vi "Main Page.vi"(8 "error in (no error)":errorcluster, 11 "Node Ptr":T3 format="%.0x") -> (0 "error out":errorcluster)   [LabVIEW 2020, in "Instrument Addon System Explorer.lvlib"]
uses:
  Instrument Addon System Explorer.lvlib
  <vilib>/NI VeriStand/Custom Device API/Custom Device Item Ref.ctl
  Addon Shared/Types/FG Control.ctl
  <vilib>/NI/NI VeriStand Hardware Resource Discovery/_Types/Filter Type.ctl
  <vilib>/NI/NI VeriStand Advanced SysDef API/SysDef API/SysDef.Property.Get.vi
  <vilib>/NI/NI VeriStand Advanced SysDef API/_SubVIs/SysDef.Property.Get.String.vi
  <vilib>/NI/NI VeriStand Advanced SysDef API/SysDef API/SysDef.Property.Set.vi
  <vilib>/NI/NI VeriStand Advanced SysDef API/_SubVIs/SysDef.Property.Set.String.vi
  <vilib>/NI VeriStand/Custom Device API/NI VeriStand - Get Item Property.vi
  <vilib>/NI VeriStand/Custom Device API/Get Item Property (Boolean).vi
  <vilib>/NI VeriStand/Custom Device API/Get Item Property (U32).vi
  <vilib>/NI VeriStand/Custom Device API/Get Item Property (String).vi
  <vilib>/NI VeriStand/Custom Device API/NI VeriStand - Set Item Property.vi
  <vilib>/NI VeriStand/Custom Device API/Set Item Property (Boolean).vi
  <vilib>/NI VeriStand/Custom Device API/Set Item Property (U32).vi
  <vilib>/NI VeriStand/Custom Device API/Set Item Property (String).vi
  <vilib>/Utility/LVClass/Get LV Class Default Value.vi
  Includes/Protocols.lvlibp/Protocol Parent/Protocol Parent.lvclass
  <vilib>/NI VeriStand/Custom Device API/Custom Device API.lvlib
  Addon Shared/Instrument Addon Shared.lvlib
  <vilib>/NI/NI VeriStand Hardware Resource Discovery/NIVS Hardware Discovery.lvlib
  APIs/Scripting API/Instrument Addon Scripting API.lvlib
panel:
  out "Version":string
  in  "PCL Decimation":u32=1 min=1 max=10000 step=1
  in  "Protocol Settings":T1(tab)=enum."TCP/IP"
  in  "COM Browse":bool
  in  "Termination Character":u8=10 format="%.0x"
  in  "End Write":bool=TRUE caption="End Write on Termination Character?"
  in  "End Read":bool=TRUE caption="End Read on Termination Character?"
  in  "XOFF":T2(ring)=enum."DC3"
  in  "XON":T2(ring)=enum."DC1"
  in  "Flow Control":u16(ring) items=["None"=0, "XON/XOFF"=1, "RTS/CTS"=2, "DTR/DSR"=4]
  in  "Stop Bits":u16(ring)=10 items=["1.0"=10, "1.5"=15, "2.0"=20]
  in  "Parity":enum16{"None", "Odd", "Even", "Mark", "Space"}(ring)
  in  "Data Bits":u16=8 min=5 max=8 step=1
  in  "Baud Rate":u32(ring)=9600 items=["75"=75, "110"=110, "134"=134, "150"=150, "300"=300, "600"=600, "1200"=1200, "1800"=1800, "2400"=2400, "4800"=4800, "7200"=7200, "9600"=9600, "14400"=14400, "19200"=19200, "28800"=28800, "38400"=38400, "56000"=56000, "57600"=57600, "115200"=115200, "128000"=128000, "230400"=230400, "460800"=460800, "921600"=921600, "1843200"=1843200, "3000000"=3000000]
  in  "Port":string="COM1"
  in  "VISA Browse":bool
  in  "Append Write Termination Character":bool caption="Append Write Termination Character?"
  in  "Timeout":u32=2000 caption="Timeout (ms)"
  in  "Termination Character":u8=10 format="%.0x"
  in  "Enable Termination Character":bool=TRUE caption="Enable Termination Character?"
  in  "VISA Resource":string="GPIB0::2::INSTR"
  in  "Port":u16
  in  "IP Address":string="localhost"
  in  "UDP Browse":bool
  in  "Target Port":u16
  in  "Target IP Address":string="localhost"
  in  "Local Port":u16
  in  "Local IP Address":string="localhost"
  in  "Assert REN w/ IFC":bool=TRUE caption="Assert REN w/ IFC?"
  in  "IST Bit Sense":bool=TRUE caption="IST Bit Sense?"
  in  "System Controller":bool=TRUE caption="System Controller?"
  in  "GPIB Address":string="1"
  in  "ConvBox Address":string="0"
  in  "ConvBox Browse":bool
  in  "ConvBox Port":string="COM1"
  in  "Protocol":string(combo)
  in  "SHDocVw.IWebBrowser":refnum<k7>(container)
  in  "Header":cluster{"Section Name":string}={"Section Name"="Addon Settings"}
  in  "Description":string
  in  "Name":string
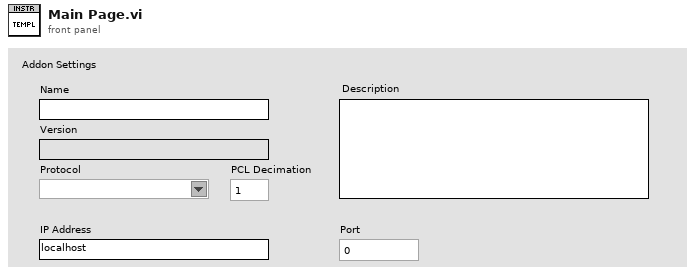
[diagram p1: front panel]
types:
  T1 = enum32{"RS232", "VISA", "TCP/IP", "UDP", "ConvBox"}
  T2 = enum16{"NUL", "SOH", "STX", "ETX", "EOT", "ENQ", "ACK", "BEL", "BS", "HT", "LF", "VT", "FF", "CR", "SO", "SI", "DLE", "DC1", "DC2", "DC3", "DC4", "NAK", "SYN", "ETB", "CAN", "EM", "SUB", "ESC", "FS", "GS", "RS", "US", "SP", "!", "\"", "#", "$", "%", "&", "'", "(", ")", "*", "+", ",", "- (-)", ".", "/", "0", "1", "2", "3", "4", "5", "6", "7", "8", "9", ":", ";", "<", "=", ">", "?", "@", "A", "B", "C", "D", "E", "F", "G", "H", "I", "J", "K", "L", "M", "N", "O", "P", "Q", "R", "S", "T", "U", "V", "W", "X", "Y", "Z", "[", "\\", "]", "^", "_", "`", "a", "b", "c", "d", "e", "f", "g", "h", "i", "j", "k", "l", "m", "n", "o", "p", "q", "r", "s", "t", "u", "v", "w", "x", "y", "z", "{", "|", "}", "~"}
  T3 = typedef "Custom Device API.lvlib/Custom Device Item Ref.ctl" = u64
  T4 = typedef "Instrument Addon Shared.lvlib/FG Control.ctl" = enum16{"Get", "Set"}
  T5 = typedef "NIVS Hardware Discovery.lvlib/Filter Type.ctl" = enum16{"Device Category", "Product Name", "Ethernet", "XNET", "VISA", "FPGA", "EtherCAT Master", "DAQmx", "GPIB", "Serial"}
  T6 = typedef "Custom Device API.lvlib/Custom Device Commands.ctl" = enum16{"Default", "Item renamed", "Shutdown", "Dynamic button pressed"}
  T7 = typedef "Instrument Addon Shared.lvlib/VISA Settings.ctl" = cluster{"VISA Resource":string, "Enable Termination Character":bool, "Termination Character":u8, "Timeout":u32, "Append Write Termination Character":bool}
  T8 = typedef "Instrument Addon Shared.lvlib/TCPIP Settings.ctl" = cluster{"IP Address":string, "Port":u16}
  T9 = typedef "Instrument Addon Shared.lvlib/UDP Settings.ctl" = cluster{"Local IP Address":string, "Local Port":u16, "Target IP Address":string, "Target Port":u16}
  T10 = typedef "Instrument Addon Shared.lvlib/RSXXX Port Settings.ctl" = cluster{"Port":string, "Baud Rate":u32, "Data Bits":u16, "Parity":enum16{"None", "Odd", "Even", "Mark", "Space"}, "Stop Bits":u16, "Flow Control":u16, "XON":enum16{"NUL", "SOH", "STX", "ETX", "EOT", "ENQ", "ACK", "BEL", "BS", "HT", "LF", "VT", "FF", "CR", "SO", "SI", "DLE", "DC1", "DC2", "DC3", "DC4", "NAK", "SYN", "ETB", "CAN", "EM", "SUB", "ESC", "FS", "GS", "RS", "US", "SP", "!", "\"", "#", "$", "%", "&", "'", "(", ")", "*", "+", ",", "- (-)", ".", "/", "0", "1", "2", "3", "4", "5", "6", "7", "8", "9", ":", ";", "<", "=", ">", "?", "@", "A", "B", "C", "D", "E", "F", "G", "H", "I", "J", "K", "L", "M", "N", "O", "P", "Q", "R", "S", "T", "U", "V", "W", "X", "Y", "Z", "[", "\\", "]", "^", "_", "`", "a", "b", "c", "d", "e", "f", "g", "h", "i", "j", "k", "l", "m", "n", "o", "p", "q", "r", "s", "t", "u", "v", "w", "x", "y", "z", "{", "|", "}", "~"}, "XOFF":enum16{"NUL", "SOH", "STX", "ETX", "EOT", "ENQ", "ACK", "BEL", "BS", "HT", "LF", "VT", "FF", "CR", "SO", "SI", "DLE", "DC1", "DC2", "DC3", "DC4", "NAK", "SYN", "ETB", "CAN", "EM", "SUB", "ESC", "FS", "GS", "RS", "US", "SP", "!", "\"", "#", "$", "%", "&", "'", "(", ")", "*", "+", ",", "- (-)", ".", "/", "0", "1", "2", "3", "4", "5", "6", "7", "8", "9", ":", ";", "<", "=", ">", "?", "@", "A", "B", "C", "D", "E", "F", "G", "H", "I", "J", "K", "L", "M", "N", "O", "P", "Q", "R", "S", "T", "U", "V", "W", "X", "Y", "Z", "[", "\\", "]", "^", "_", "`", "a", "b", "c", "d", "e", "f", "g", "h", "i", "j", "k", "l", "m", "n", "o", "p", "q", "r", "s", "t", "u", "v", "w", "x", "y", "z", "{", "|", "}", "~"}, "End Read on Termination Character":bool, "End Write on Termination Character":bool, "Termination Character":u8}
  T11 = typedef "Instrument Addon Shared.lvlib/GPIB ConvBox Settings.ctl" = cluster{"Port":string, "ConvBox Address":string, "Assert Ren with IFC":bool, "System controller":bool, "IST bit sense":bool, "GPIB Address":string}
  T12 = typedef "Protocols.lvlibp/Protocol Parent.lvclass/Base Protocol Type.ctl" = enum16{"RS-XXX", "VISA", "TCPIP", "UDP", "GPIB ConvBox"}
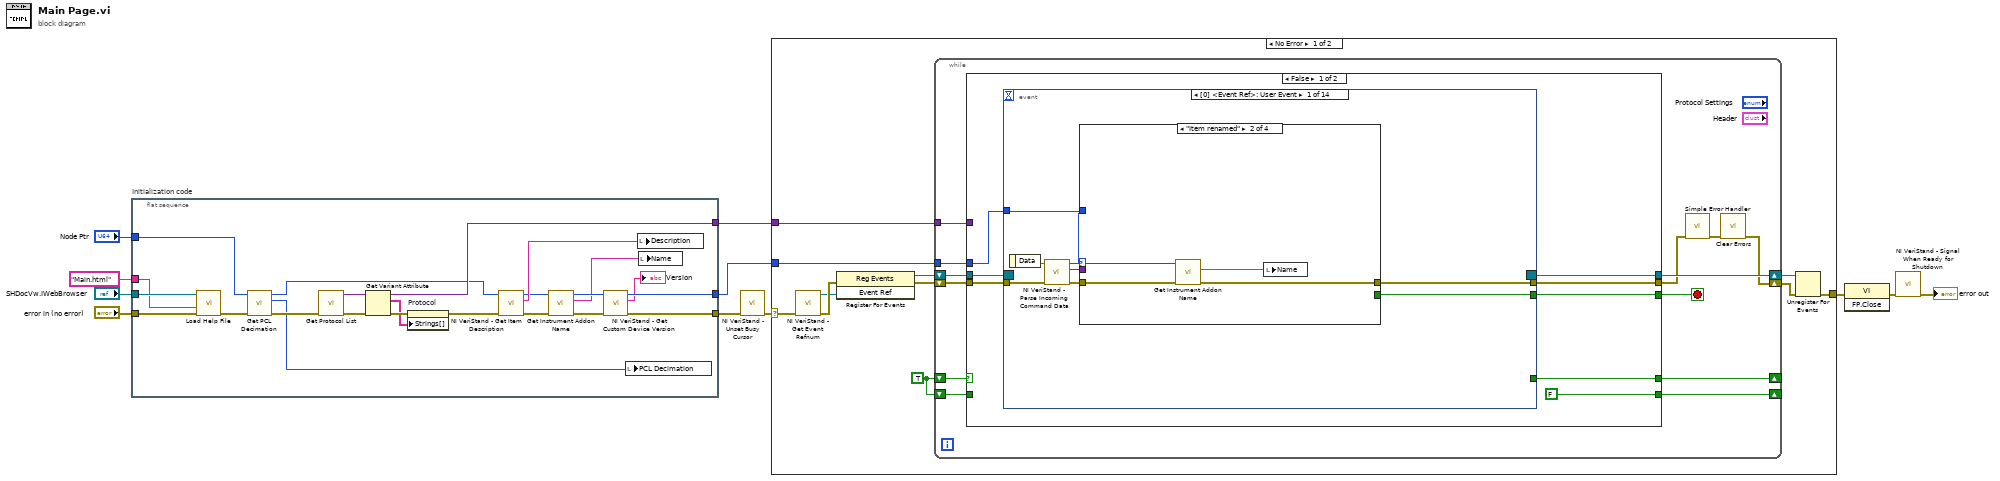
[diagram p0: block diagram]
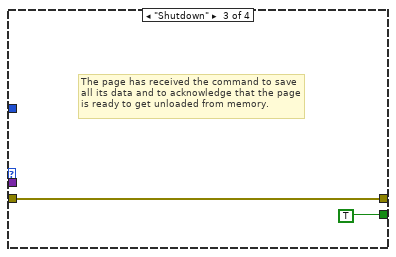
[diagram p3: hidden frame]
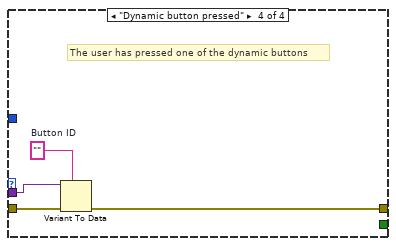
[diagram p4: hidden frame]
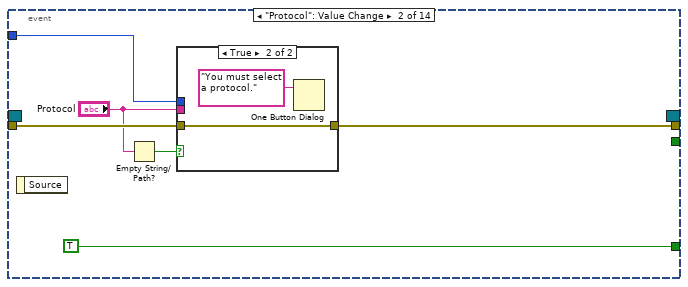
[diagram p5: hidden frame]
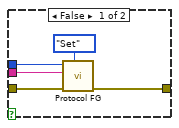
[diagram p6: hidden frame]
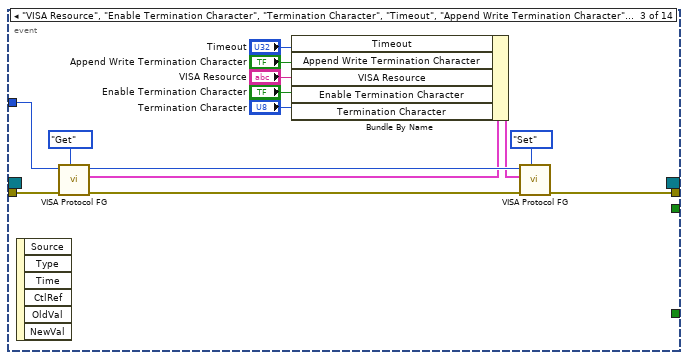
[diagram p7: hidden frame]
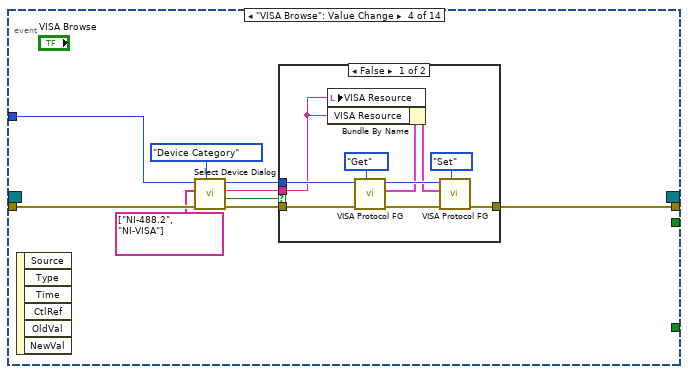
[diagram p8: hidden frame]
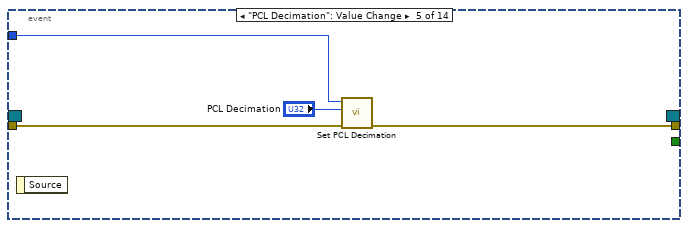
[diagram p10: hidden frame]
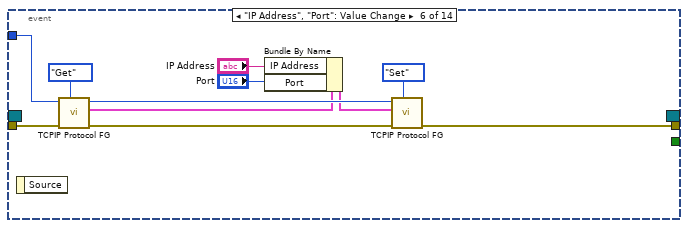
[diagram p11: hidden frame]
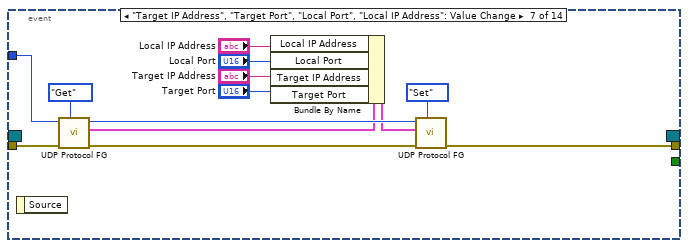
[diagram p12: hidden frame]
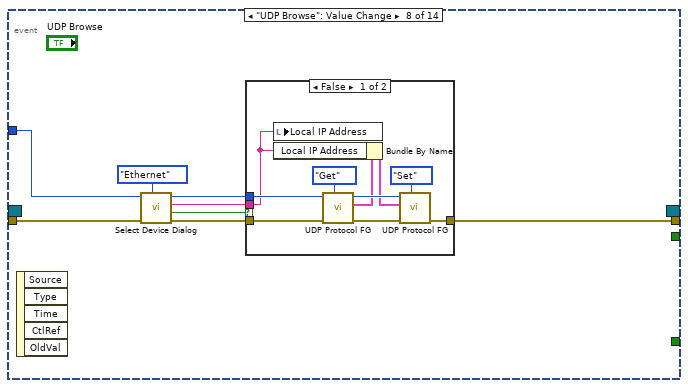
[diagram p13: hidden frame]
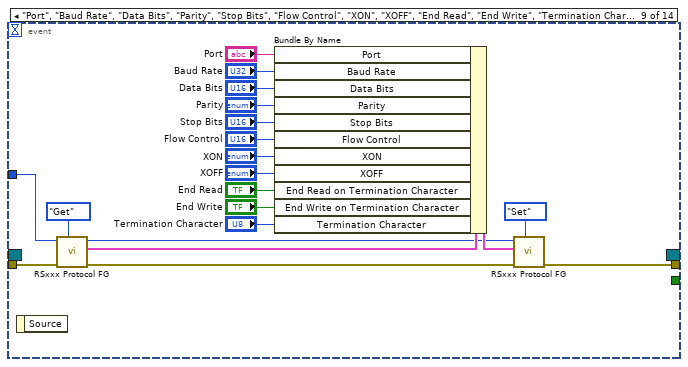
[diagram p15: hidden frame]
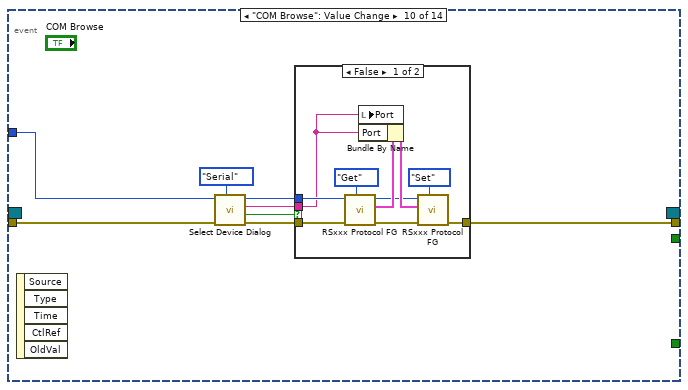
[diagram p16: hidden frame]
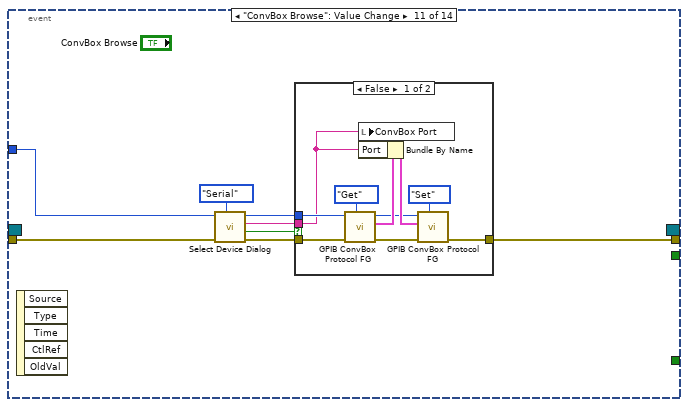
[diagram p18: hidden frame]
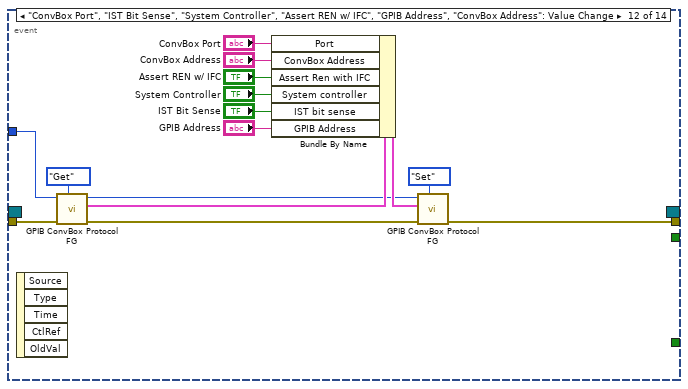
[diagram p20: hidden frame]
diagram:
  n1 = flat-sequence "Initialization code" {
    tunnel: "error in (no error)" -> [w33]
    tunnel: "Node Ptr" -> [w19]
    tunnel: [w24] -> w7
    tunnel: [w23] -> w4
    tunnel: "SHDocVw.IWebBrowser" -> [w32]
    tunnel: "Main.html" ("HTML File") -> [w31]
    tunnel: [w26] -> w1
    frame #0 {
      n2 = call "Load Help File.vi"("error in (no error)"=w33, "HTML File to Load"=w31, "SHDocVw.IWebBrowser2"=w32) -> ("error out"=w21:errorcluster)  [unwired: 8 in]
      n3 = call "Get PCL Decimation.vi"("error in (no error)"=w21, "instrument addon refnum in"=w19) -> ("error out"=w20:errorcluster, "PCL decimation"=w17:u32, "instrument addon refnum out"=w18:T3)  [unwired: 7 in]
      n4 = call "Get Protocol List.vi"("error in (no error)"=w20) -> ("error out"=w29:errorcluster, "Class Lookup"=w30:variant)  [unwired: 9 in]
      n5 = Get Variant Attribute(Variant=w30, error in=w29) -> (duplicate Variant=w26:variant, names=w27:string[], error out=w28:errorcluster)  [unwired: 2 in, 1 out]
      n6 = property on="Protocol" class="CmbBox"(error in=w28, "Strings[]"=w27) -> (error out=w25:errorcluster)  [unwired: 1 in, 1 out]
      n7 = call <vilib>:"NI VeriStand - Get Item Description.vi"("error in (no error)"=w25, "Item Ref in"=w18) -> ("error out"=w16:errorcluster, "Description"=w34:string, "Item Ref out"=w14:T3)  [unwired: 7 out]
      n8 = call "Get Instrument Addon Name.vi"("error in (no error)"=w16, "instrument addon refnum in"=w14) -> ("error out"=w15:errorcluster, "name"=w12:string, "instrument addon refnum out"=w13:T3)  [unwired: 7 in]
      n9 = call <vilib>:"NI VeriStand - Get Custom Device Version.vi"("error in (no error)"=w15, "Device Ref in"=w13) -> ("error out"=w24:errorcluster, "Value"=→"Version":string, "Device Ref out"=w23:T3)  [unwired: 7 in]
      n10 = local write "PCL Decimation"(w17) -> ()
      n11 = local write "Description"(w34) -> ()
      n12 = local write "Name"(w12) -> ()
    }
  }
  n13 = call <vilib>:"NI VeriStand - Unset Busy Cursor.vi"("error in (no error)"=w7) -> ("error out"=w6:errorcluster)  [unwired: 10 out]
  n14 = case shown="No Error" w6 {
    selector: w6 -> [w37 w343]
    tunnel: [w42 w341] -> w11
    tunnel: w4 -> [w38 _]
    tunnel: w1 -> [w36 _]
    frame No Error {
      w35 = TRUE
      n15 = call <vilib>:"NI VeriStand - Get Event Refnum.vi"("error in (no error)"=w37) -> ("error out"=w45:errorcluster, "Event Ref"=w41:refnum<user-event>)  [unwired: 9 out]
      n16 = register-events(error in=w45, w41) -> (reference out=w39:refnum<event-registration>, error out=w40:errorcluster)  [unwired: 1 in]
      n17 = while {
        tunnel: w38 -> [w54]
        shift-right: [w51] -> w43
        shift-left: w40 -> [w57]
        shift-right: [w58] -> w44
        shift-left: w39 -> [w56]
        tunnel: w36 -> [w50]
        shift-right: [w48] -> _
        shift-left: w35 -> [w49]
        shift-right: [w46] -> _
        shift-left: w35 -> [w47]
        stop <- w55 stop-if-true
        n18 = case shown="False" w49 {
          tunnel: [w66 w268] -> w58
          tunnel: w57 -> [w65 w276]
          tunnel: w56 -> [w64 w268]
          tunnel: [w63 _] -> w55
          tunnel: w54 -> [w62 w275]
          tunnel: [w61 w263] -> w53
          tunnel: w50 -> [_ w273]
          tunnel: [w60 w261] -> w48
          tunnel: w47 -> [_ w262]
          tunnel: [FALSE w261] -> w46
          frame False {
            n19 = event shown="[0] <Event Ref>: User Event" {
              selector: w64 -> [_ _ _ _ _ _ _ _ _ _ _ _ _ _]
              dyn-events: [_ _ _ _ _ _ _ _ _ _ _ _ _ _] -> w66
              timeout: _ -> [_ _ _ _ _ _ _ _ _ _ _ _ _ _]
              tunnel: w65 -> [w74 w90 w111 w120 w136 w146 w159 w167 w196 w206 w225 w245 w256 w259]
              tunnel: [w70 _ _ _ _ _ _ _ _ _ _ _ _ _] -> w63
              tunnel: [w69 w86 w107 w121 w135 w142 w155 w168 w198 w207 w226 w252 w255 w258] -> w61
              tunnel: w62 -> [w68 w91 w110 w118 w133 w145 w158 w165 w194 w205 w224 w244 w253 w260]
              tunnel: [_ TRUE _ _ _ _ _ _ _ _ _ _ _ _] -> w60
              event User Event {
                n20 = event-data() -> ("Data"=w73:string)  [unwired: 1 out]
                n21 = call <vilib>:"NI VeriStand - Parse Incoming Command Data.vi"("error in (no error)"=w74, "Incoming data"=w73) -> ("error out"=w72:errorcluster, "Outgoing data"=w67:variant, "Action"=w71:T6)  [unwired: 7 out]
                n22 = case shown="\"Item renamed\"" w71 {
                  tunnel: w72 -> [w75 w77 w80 w85]
                  tunnel: [_ _ TRUE _] -> w70
                  tunnel: [w75 w76 w80 w82] -> w69
                  tunnel: w68 -> [_ w78 _ _]
                  tunnel: w67 -> [_ _ _ w84]
                  frame "Default", Default {
                  }
                  frame "Item renamed" {
                    n23 = call "Get Instrument Addon Name.vi"("error in (no error)"=w77, "instrument addon refnum in"=w78) -> ("error out"=w76:errorcluster, "name"=w79:string)  [unwired: 7 in, 1 out]
                    n24 = local write "Name"(w79) -> ()
                  }
                  frame "Shutdown" {
                    # "The page has received the command to save all its data and to acknowledge that the page is ready to get unloaded from memory."
                  }
                  frame "Dynamic button pressed" {
                    w83 = ""  # Button ID
                    # "The user has pressed one of the dynamic buttons"
                    n25 = Variant To Data(error in=w85, type=w83, Variant=w84) -> (error out=w82:errorcluster)  [unwired: 1 out]
                  }
                }
              }
              event "Protocol": Value Change {
                n26 = event-data() -> ()  [unwired: 2 out]
                n27 = Empty String/Path?(string/path="Protocol") -> (empty?=w88:bool)
                n28 = case shown="True" w88 {
                  tunnel: w91 -> [w94 _]
                  tunnel: w90 -> [w95 w97]
                  tunnel: [w92 w97] -> w86
                  tunnel: "Protocol" -> [w93 _]
                  frame False {
                    n29 = call "Protocol FG.vi"("Action"=FG_Control."Set", "error in (no error)"=w95, "Protocol"=w93, "Device Item Ref in"=w94) -> ("error out"=w92:errorcluster)  [unwired: 5 in, 2 out]
                  }
                  frame True {
                    n30 = One Button Dialog(message="You must select a protocol.") -> ()  [unwired: 1 in, 1 out]
                  }
                }
              }
              event "VISA Resource", "Enable Termination Character", "Termination Character", "Timeout", "Append Write Termination Character": Value Change {
                n31 = event-data() -> ()  [unwired: 7 out]
                n32 = call "VISA Protocol FG.vi"("Action"=FG_Control."Get", "error in (no error)"=w111, "Device Item Ref in"=w110) -> ("error out"=w108:errorcluster, "VISA Config"=w105:T7, "Item Ref out"=w106:T3)  [unwired: 6 in]
                n33 = Bundle By Name(cluster=w105, "Timeout"="Timeout", "Append Write Termination Character"="Append Write Termination Character", "VISA Resource"="VISA Resource", "Enable Termination Character"="Enable Termination Character", "Termination Character"="Termination Character") -> (w104:T7)
                n34 = call "VISA Protocol FG.vi"("Action"=FG_Control."Set", "error in (no error)"=w108, "VISA Config"=w104, "Device Item Ref in"=w106) -> ("error out"=w107:errorcluster)  [unwired: 5 in, 2 out]
              }
              event "VISA Browse": Value Change {
                n35 = event-data() -> ()  [unwired: 7 out]
                n36 = call <vilib>:"Select Device Dialog.vi"("Filter Type"=Filter_Type."Device Category", "error in (no error)"=w120, "Filter Names"=string[] ["NI-488.2", "NI-VISA"], "Item Ref in"=w118) -> ("error out"=w119:errorcluster, "Cancelled?"=w116:bool, "Selected Alias"=w115:string, "Item Ref out"=w117:T3)  [unwired: 4 in]
                n37 = case shown="False" w116 {
                  tunnel: w119 -> [w130 w132]
                  tunnel: w117 -> [w129 _]
                  tunnel: [w126 w132] -> w121
                  tunnel: w115 -> [w122 _]
                  frame False {
                    n38 = local write "VISA Resource"(w122) -> ()
                    n39 = call "VISA Protocol FG.vi"("Action"=FG_Control."Get", "error in (no error)"=w130, "Device Item Ref in"=w129) -> ("error out"=w127:errorcluster, "VISA Config"=w124:T7, "Item Ref out"=w125:T3)  [unwired: 6 in]
                    n40 = Bundle By Name(cluster=w124, "VISA Resource"=w122) -> (w123:T7)
                    n41 = call "VISA Protocol FG.vi"("Action"=FG_Control."Set", "error in (no error)"=w127, "VISA Config"=w123, "Device Item Ref in"=w125) -> ("error out"=w126:errorcluster)  [unwired: 5 in, 2 out]
                  }
                  frame True {
                  }
                }
              }
              event "PCL Decimation": Value Change {
                n42 = event-data() -> ()  [unwired: 2 out]
                n43 = call "Set PCL Decimation.vi"("error in (no error)"=w136, "PCL decimation"="PCL Decimation", "instrument addon refnum in"=w133) -> ("error out"=w135:errorcluster)  [unwired: 7 in, 1 out]
              }
              event "IP Address", "Port": Value Change {
                n44 = event-data() -> ()  [unwired: 2 out]
                n45 = call "TCPIP Protocol FG.vi"("Action"=FG_Control."Get", "error in (no error)"=w146, "Device Item Ref in"=w145) -> ("error out"=w143:errorcluster, "TCP/IP Config"=w140:T8, "Item Ref out"=w141:T3)  [unwired: 6 in]
                n46 = Bundle By Name(cluster=w140, "IP Address"="IP Address", "Port"="Port") -> (w139:T8)
                n47 = call "TCPIP Protocol FG.vi"("Action"=FG_Control."Set", "error in (no error)"=w143, "TCP/IP Config"=w139, "Device Item Ref in"=w141) -> ("error out"=w142:errorcluster)  [unwired: 5 in, 2 out]
              }
              event "Target IP Address", "Target Port", "Local Port", "Local IP Address": Value Change {
                n48 = event-data() -> ()  [unwired: 2 out]
                n49 = call "UDP Protocol FG.vi"("Action"=FG_Control."Get", "error in (no error)"=w159, "Device Item Ref in"=w158) -> ("error out"=w156:errorcluster, "UDP Config"=w153:T9, "Item Ref out"=w154:T3)  [unwired: 6 in]
                n50 = Bundle By Name(cluster=w153, "Local IP Address"="Local IP Address", "Local Port"="Local Port", "Target IP Address"="Target IP Address", "Target Port"="Target Port") -> (w152:T9)
                n51 = call "UDP Protocol FG.vi"("Action"=FG_Control."Set", "error in (no error)"=w156, "UDP Config"=w152, "Device Item Ref in"=w154) -> ("error out"=w155:errorcluster)  [unwired: 5 in, 2 out]
              }
              event "UDP Browse": Value Change {
                n52 = event-data() -> ()  [unwired: 6 out]
                n53 = call <vilib>:"Select Device Dialog.vi"("Filter Type"=Filter_Type."Ethernet", "error in (no error)"=w167, "Item Ref in"=w165) -> ("error out"=w166:errorcluster, "Cancelled?"=w163:bool, "Selected Alias"=w162:string, "Item Ref out"=w164:T3)  [unwired: 5 in]
                n54 = case shown="False" w163 {
                  tunnel: w166 -> [w177 w179]
                  tunnel: w164 -> [w176 _]
                  tunnel: [w173 w179] -> w168
                  tunnel: w162 -> [w169 _]
                  frame False {
                    n55 = local write "Local IP Address"(w169) -> ()
                    n56 = call "UDP Protocol FG.vi"("Action"=FG_Control."Get", "error in (no error)"=w177, "Device Item Ref in"=w176) -> ("error out"=w174:errorcluster, "UDP Config"=w171:T9, "Item Ref out"=w172:T3)  [unwired: 6 in]
                    n57 = Bundle By Name(cluster=w171, "Local IP Address"=w169) -> (w170:T9)
                    n58 = call "UDP Protocol FG.vi"("Action"=FG_Control."Set", "error in (no error)"=w174, "UDP Config"=w170, "Device Item Ref in"=w172) -> ("error out"=w173:errorcluster)  [unwired: 5 in, 2 out]
                  }
                  frame True {
                  }
                }
              }
              event "Port", "Baud Rate", "Data Bits", "Parity", "Stop Bits", "Flow Control", "XON", "XOFF", "End Read", "End Write", "Termination Character": Value Change {
                n59 = event-data() -> ()  [unwired: 2 out]
                n60 = call "RSxxx Protocol FG.vi"("Action"=FG_Control."Get", "error in (no error)"=w196, "Device Item Ref in"=w194) -> ("error out"=w195:errorcluster, "Serial Config"=w193:T10, "Item Ref out"=w180:T3)  [unwired: 6 in]
                n61 = Bundle By Name(cluster=w193, "Port"="Port", "Baud Rate"="Baud Rate", "Data Bits"="Data Bits", "Parity"="Parity", "Stop Bits"="Stop Bits", "Flow Control"="Flow Control", "XON"="XON", "XOFF"="XOFF", "End Read on Termination Character"="End Read", "End Write on Termination Character"="End Write", "Termination Character"="Termination Character") -> (w192:T10)
                n62 = call "RSxxx Protocol FG.vi"("Action"=FG_Control."Set", "error in (no error)"=w195, "Serial Config"=w192, "Device Item Ref in"=w180) -> ("error out"=w198:errorcluster)  [unwired: 5 in, 2 out]
              }
              event "COM Browse": Value Change {
                n63 = event-data() -> ()  [unwired: 6 out]
                n64 = call <vilib>:"Select Device Dialog.vi"("Filter Type"=Filter_Type."Serial", "error in (no error)"=w206, "Item Ref in"=w205) -> ("error out"=w203:errorcluster, "Cancelled?"=w202:bool, "Selected Alias"=w201:string, "Item Ref out"=w204:T3)  [unwired: 5 in]
                n65 = case shown="False" w202 {
                  tunnel: [w216 w218] -> w207
                  tunnel: w203 -> [w214 w218]
                  tunnel: w204 -> [w212 _]
                  tunnel: w201 -> [w208 _]
                  frame False {
                    n66 = call "RSxxx Protocol FG.vi"("Action"=FG_Control."Get", "error in (no error)"=w214, "Device Item Ref in"=w212) -> ("error out"=w213:errorcluster, "Serial Config"=w211:T10, "Item Ref out"=w209:T3)  [unwired: 6 in]
                    n67 = local write "Port"(w208) -> ()
                    n68 = Bundle By Name(cluster=w211, "Port"=w208) -> (w210:T10)
                    n69 = call "RSxxx Protocol FG.vi"("Action"=FG_Control."Set", "error in (no error)"=w213, "Serial Config"=w210, "Device Item Ref in"=w209) -> ("error out"=w216:errorcluster)  [unwired: 5 in, 2 out]
                  }
                  frame True {
                  }
                }
              }
              event "ConvBox Browse": Value Change {
                n70 = event-data() -> ()  [unwired: 6 out]
                n71 = call <vilib>:"Select Device Dialog.vi"("Filter Type"=Filter_Type."Serial", "error in (no error)"=w225, "Item Ref in"=w224) -> ("error out"=w222:errorcluster, "Cancelled?"=w221:bool, "Selected Alias"=w220:string, "Item Ref out"=w223:T3)  [unwired: 5 in]
                n72 = case shown="False" w221 {
                  tunnel: [w235 w237] -> w226
                  tunnel: w222 -> [w233 w237]
                  tunnel: w223 -> [w231 _]
                  tunnel: w220 -> [w227 _]
                  frame False {
                    n73 = call "GPIB ConvBox Protocol FG.vi"("Action"=FG_Control."Get", "error in (no error)"=w233, "Device Item Ref in"=w231) -> ("error out"=w232:errorcluster, "GPIB ConvBox Config"=w230:T11, "Item Ref out"=w228:T3)  [unwired: 6 in]
                    n74 = local write "ConvBox Port"(w227) -> ()
                    n75 = Bundle By Name(cluster=w230, "Port"=w227) -> (w229:T11)
                    n76 = call "GPIB ConvBox Protocol FG.vi"("Action"=FG_Control."Set", "error in (no error)"=w232, "GPIB ConvBox Config"=w229, "Device Item Ref in"=w228) -> ("error out"=w235:errorcluster)  [unwired: 5 in, 2 out]
                  }
                  frame True {
                  }
                }
              }
              event "ConvBox Port", "IST Bit Sense", "System Controller", "Assert REN w/ IFC", "GPIB Address", "ConvBox Address": Value Change {
                n77 = event-data() -> ()  [unwired: 6 out]
                n78 = call "GPIB ConvBox Protocol FG.vi"("Action"=FG_Control."Get", "error in (no error)"=w245, "Device Item Ref in"=w244) -> ("error out"=w249:errorcluster, "GPIB ConvBox Config"=w248:T11, "Item Ref out"=w246:T3)  [unwired: 6 in]
                n79 = Bundle By Name(cluster=w248, "Port"="ConvBox Port", "ConvBox Address"="ConvBox Address", "Assert Ren with IFC"="Assert REN w/ IFC", "System controller"="System Controller", "IST bit sense"="IST Bit Sense", "GPIB Address"="GPIB Address") -> (w247:T11)
                n80 = call "GPIB ConvBox Protocol FG.vi"("Action"=FG_Control."Set", "error in (no error)"=w249, "GPIB ConvBox Config"=w247, "Device Item Ref in"=w246) -> ("error out"=w252:errorcluster)  [unwired: 5 in, 2 out]
              }
              event "Name": Value Change {
                n81 = event-data() -> ()  [unwired: 2 out]
                n82 = call "Set Instrument Addon Name.vi"("error in (no error)"=w256, "name"="Name", "instrument addon refnum in"=w253) -> ("error out"=w255:errorcluster)  [unwired: 7 in, 1 out]
              }
              event "Description": Value Change {
                n83 = event-data() -> ()  [unwired: 2 out]
                n84 = call <vilib>:"NI VeriStand - Set Item Description.vi"("error in (no error)"=w259, "Description"="Description", "Item Ref in"=w260) -> ("error out"=w258:errorcluster)  [unwired: 8 out]
              }
            }
          }
          frame True {
            w261 = FALSE
            n85 = call "Protocol FG.vi"("Action"=FG_Control."Get", "error in (no error)"=w276, "Device Item Ref in"=w275) -> ("error out"=w272:errorcluster, "Protocol out"=w269:string, "Item Ref out"=w271:T3)  [unwired: 6 in]
            n86 = call "Lookup Base Protocol Class and Info.vi"("error in (no error)"=w272, "Protocol in"=w269, "Class Lookup"=w273) -> ("error out"=w274:errorcluster, "Protocol out"=w267:T12, "Error Codes"=w266:cluster{"Code":i32, "String":string}[])  [unwired: 4 in, 2 out]
            n87 = case shown="\"VISA\"" w267 {
              tunnel: w274 -> [w293 w301 w311 w328 w340]
              tunnel: [w292 w300 w310 w327 w339] -> w264
              tunnel: w271 -> [w291 w299 w309 w326 w338]
              tunnel: [w283 w294 w302 w312 w329] -> w265
              frame "VISA" {
                n88 = call "VISA Protocol FG.vi"("Action"=FG_Control."Get", "error in (no error)"=w293, "Device Item Ref in"=w291) -> ("error out"=w292:errorcluster, "VISA Config"=w289:T7, "Item Ref out"=w283:T3)  [unwired: 6 in]
                n89 = Unbundle By Name(w289) -> ("Append Write Termination Character"=w284:bool, "Timeout"=w285:u32, "VISA Resource"=w288:string, "Enable Termination Character"=w287:bool, "Termination Character"=w286:u8)
                n90 = local write "Append Write Termination Character"(w284) -> ()
                n91 = local write "Enable Termination Character"(w287) -> ()
                n92 = local write "Termination Character"(w286) -> ()
                n93 = local write "Timeout"(w285) -> ()
                n94 = local write "VISA Resource"(w288) -> ()
              }
              frame "TCPIP" {
                n95 = call "TCPIP Protocol FG.vi"("Action"=FG_Control."Get", "error in (no error)"=w301, "Device Item Ref in"=w299) -> ("error out"=w300:errorcluster, "TCP/IP Config"=w297:T8, "Item Ref out"=w294:T3)  [unwired: 6 in]
                n96 = Unbundle By Name(w297) -> ("IP Address"=w296:string, "Port"=w295:u16)
                n97 = local write "IP Address"(w296) -> ()
                n98 = local write "Port"(w295) -> ()
              }
              frame "UDP" {
                n99 = call "UDP Protocol FG.vi"("Action"=FG_Control."Get", "error in (no error)"=w311, "Device Item Ref in"=w309) -> ("error out"=w310:errorcluster, "UDP Config"=w307:T9, "Item Ref out"=w302:T3)  [unwired: 6 in]
                n100 = Unbundle By Name(w307) -> ("Local IP Address"=w306:string, "Local Port"=w305:u16, "Target IP Address"=w304:string, "Target Port"=w303:u16)
                n101 = local write "Local IP Address"(w306) -> ()
                n102 = local write "Local Port"(w305) -> ()
                n103 = local write "Target IP Address"(w304) -> ()
                n104 = local write "Target Port"(w303) -> ()
              }
              frame "RS-XXX" {
                n105 = call "RSxxx Protocol FG.vi"("Action"=FG_Control."Get", "error in (no error)"=w328, "Device Item Ref in"=w326) -> ("error out"=w327:errorcluster, "Serial Config"=w324:T10, "Item Ref out"=w312:T3)  [unwired: 6 in]
                n106 = Unbundle By Name(w324) -> ("Port"=w323:string, "Baud Rate"=w322:u32, "Data Bits"=w313:u16, "Parity"=w314:enum16{"None", "Odd", "Even", "Mark", "Space"}, "Stop Bits"=w315:u16, "Flow Control"=w316:u16, "XON"=w317:T2, "XOFF"=w318:T2, "End Read on Termination Character"=w319:bool, "End Write on Termination Character"=w320:bool, "Termination Character"=w321:u8)
                n107 = local write "Termination Character"(w321) -> ()
                n108 = local write "Flow Control"(w316) -> ()
                n109 = local write "Data Bits"(w313) -> ()
                n110 = local write "Stop Bits"(w315) -> ()
                n111 = local write "XON"(w317) -> ()
                n112 = local write "End Write"(w320) -> ()
                n113 = local write "Port"(w323) -> ()
                n114 = local write "Baud Rate"(w322) -> ()
                n115 = local write "Parity"(w314) -> ()
                n116 = local write "XOFF"(w318) -> ()
                n117 = local write "End Read"(w319) -> ()
              }
              frame "GPIB ConvBox" {
                n118 = call "GPIB ConvBox Protocol FG.vi"("Action"=FG_Control."Get", "error in (no error)"=w340, "Device Item Ref in"=w338) -> ("error out"=w339:errorcluster, "GPIB ConvBox Config"=w336:T11, "Item Ref out"=w329:T3)  [unwired: 6 in]
                n119 = Unbundle By Name(w336) -> ("Port"=w335:string, "ConvBox Address"=w334:string, "Assert Ren with IFC"=w333:bool, "System controller"=w332:bool, "IST bit sense"=w331:bool, "GPIB Address"=w330:string)
                n120 = local write "Assert REN w/ IFC"(w333) -> ()
                n121 = local write "ConvBox Port"(w335) -> ()
                n122 = local write "ConvBox Address"(w334) -> ()
                n123 = local write "System Controller"(w332) -> ()
                n124 = local write "GPIB Address"(w330) -> ()
                n125 = local write "IST Bit Sense"(w331) -> ()
              }
            }
            n126 = To Unsigned Long Integer(number=w267) -> (unsigned 32bit integer=w270:u32)
            n127 = local write "Protocol Settings"(w270) -> ()
            n128 = local write "Protocol"(w269) -> ()
            n129 = case shown="False" w262 {
              tunnel: w266 -> [w281 _]
              tunnel: w265 -> [w280 _]
              tunnel: w264 -> [w279 w282]
              tunnel: [w278 w282] -> w263
              frame False {
                n130 = call "Set Codes on all Error Channels.vi"("error in (no error)"=w279, "Error Codes"=w281, "Node Ptr in"=w280) -> ("error out"=w278:errorcluster)  [unwired: 7 in, 1 out]
              }
              frame True {
              }
            }
          }
        }
        n131 = call <vilib>:"Simple Error Handler.vi"("error in (no error)"=w53) -> ("error out"=w52:errorcluster)  [unwired: 1 in, 7 out]
        n132 = call <vilib>:"Clear Errors.vi"("error in (no error)"=w52) -> ("error out"=w51:errorcluster)  [unwired: 1 in, 5 out]
      }
      n133 = Unregister For Events(event registration refnum=w44, error in=w43) -> (error out=w42:errorcluster)
    }
    frame Error {
      n134 = call <vilib>:"Simple Error Handler.vi"("error in (no error)"=w343) -> ("error out"=w342:errorcluster)  [unwired: 1 in, 7 out]
      n135 = call <vilib>:"Clear Errors.vi"("error in (no error)"=w342) -> ("error out"=w341:errorcluster)  [unwired: 1 in, 5 out]
    }
  }
  n136 = invoke class="VI" method="FP.Close"(error in=w11) -> (error out=w10:errorcluster)  [unwired: 2 in, 2 out]
  n137 = call <vilib>:"NI VeriStand - Signal When Ready for Shutdown.vi"("error in (no error)"=w10) -> ("error out"=→"error out":errorcluster)  [unwired: 10 out]
